vi "Map Points to Origin.vi"(1 "New Origin":T2={"X"=-1, "Y"=-1}, 2 "Points":T1[](array[typedef])) -> (0 "Mapped Points":T1[](array[typedef]))   [LabVIEW 2018]
uses:
  Graham Scan Point.ctl
  Graham Scan Origin Point STYP.ctl
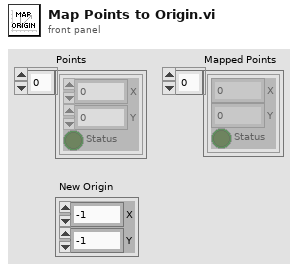
[diagram p1: front panel]
types:
  T1 = typedef "Graham Scan Point.ctl" = cluster{"X":i32, "Y":i32, "Status":bool}
  T2 = typedef "Graham Scan Origin Point STYP.ctl" = cluster{"X":i32, "Y":i32}
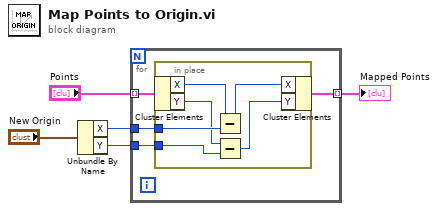
[diagram p0: block diagram]
diagram:
  n1 = Unbundle By Name("New Origin") -> ("X"=w2:i32, "Y"=w1:i32)
  n2 = for {
    tunnel: "Points" -> [w9] mode=indexing
    tunnel: [w8] -> w4 mode=indexing
    tunnel: w2 -> [w7]
    tunnel: w1 -> [w6]
    n3 = in-place {
      in-place-border: w7 -> [w14]
      in-place-border: w6 -> [w12]
      n4 = in-place-cluster #1(w9) -> ("X"=w15:i32, "Y"=w13:i32)
      n5 = Subtract(x=w15, y=w14) -> (x-y=w11:i32)
      n6 = Subtract(x=w13, y=w12) -> (x-y=w10:i32)
      n7 = in-place-cluster #1("X"=w11, "Y"=w10) -> (w8:T1)
    }
  }
  "Mapped Points" <- w4
